vi "Alarms.vi"(0 "Alarm 1":T4, 1 "Alarm 2":T4, 2 "Alarm 3":T4, 3 "Alarm 4":T4, 4 "HW CTRL Data":T2, 5 "Variables State":T3, 7 "error in (no error)":errorcluster) -> (24 "Alarms triggered?":T1, 27 "error out":errorcluster)   [LabVIEW 2014, in "SeqLoop.lvlib"]
doc: "Detecta el estado de las alarmas utilizando el Vi de \"RPNLogicSolverError\"."
uses:
  SeqLoop.lvlib
  TypeDefs/LogicParsedExpression.ctl
  TypeDefs/Variables State.ctl
  TypeDefs/HW CTRL Data.ctl
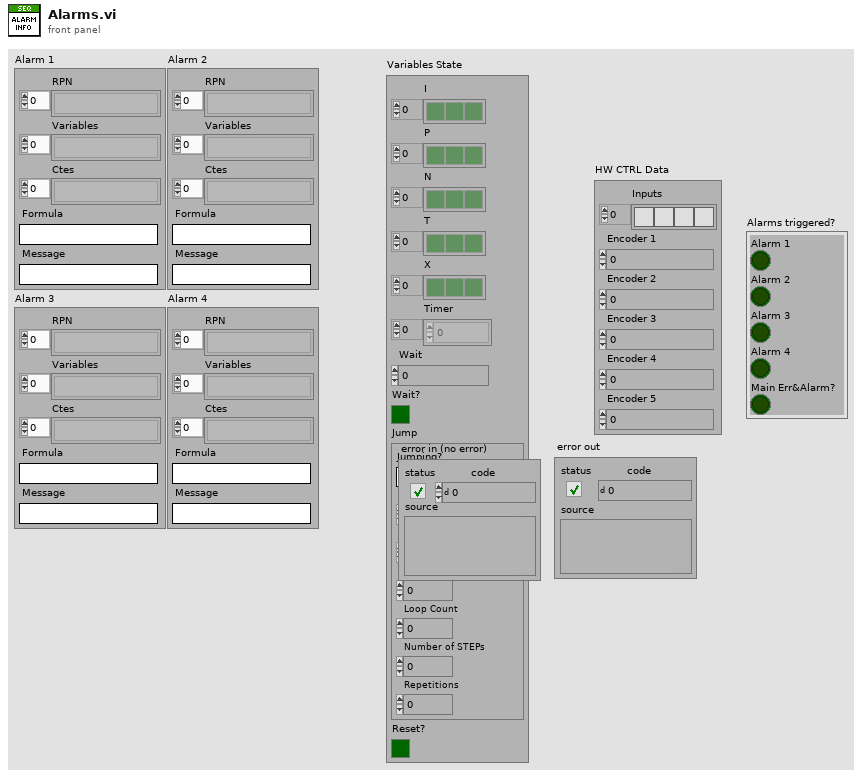
[diagram p1: front panel]
types:
  T1 = cluster{"Alarm 1":bool, "Alarm 2":bool, "Alarm 3":bool, "Alarm 4":bool, "Main Err&Alarm?":bool}
  T2 = typedef "SeqLoop.lvlib/HW CTRL Data.ctl" = cluster{"Inputs":bool[], "Encoder 1":sgl, "Encoder 2":sgl, "Encoder 3":sgl, "Encoder 4":sgl, "Encoder 5":sgl}
  T3 = typedef "SeqLoop.lvlib/Variables State.ctl" = cluster{"I":bool[], "P":bool[], "N":bool[], "T":bool[], "X":bool[], "Timer":u32[], "Wait":u32, "Wait?":bool, "Jump":cluster{"Jumping?":bool, "Previous STEP to Jump":u32, "Initial Jump STEP":u32, "STEP Count":u32, "Loop Count":u32, "Number of STEPs":u32, "Repetitions":u32}, "Reset?":bool}
  T4 = typedef "SeqLoop.lvlib/LogicParsedExpression.ctl" = cluster{"RPN ":string[], "Variables":string[], "Ctes":string[], "Formula":string, "Message":string}
  T5 = cluster{"Logic Result":bool, "Logic Result":bool, "Logic Result":bool, "Logic Result":bool, bool}
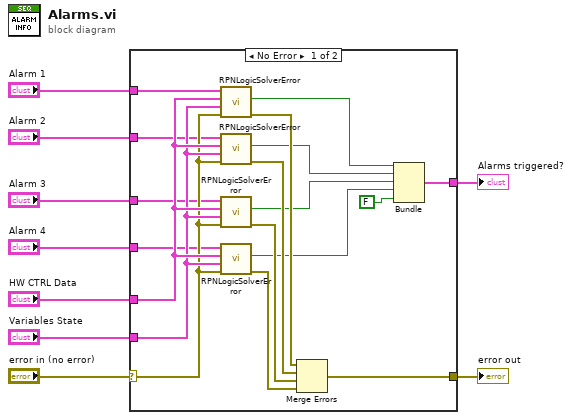
[diagram p0: block diagram]
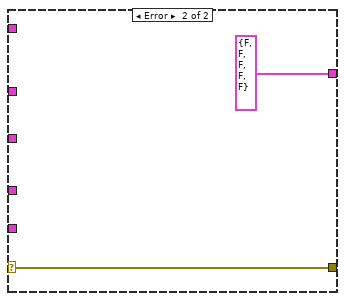
[diagram p2: hidden frame]
diagram:
  n1 = case shown="No Error" "error in (no error)" {
    selector: "error in (no error)" -> [w20 w29]
    tunnel: "Alarm 1" -> [w19 _]
    tunnel: "Alarm 2" -> [w18 _]
    tunnel: "Alarm 3" -> [w17 _]
    tunnel: "Alarm 4" -> [w16 _]
    tunnel: "HW CTRL Data" -> [w27 _]
    tunnel: "Variables State" -> [w26 _]
    tunnel: [w25 w29] -> w2
    tunnel: [w11 T5 {"Logic Result"=FALSE, "Logic Result"=FALSE, "Logic Result"=FALSE, "Logic Result"=FALSE, FALSE}] -> w1
    frame No Error {
      n2 = call "RPNLogicSolverError.vi"("error in"=w20, "Variables State in"=w26, "HW CTRL Data"=w27, "Logic Parsed Expression"=w19) -> ("error out"=w24:errorcluster, "Logic Result"=w15:bool)  [unwired: 5 in, 1 out]
      n3 = call "RPNLogicSolverError.vi"("error in"=w20, "Variables State in"=w26, "HW CTRL Data"=w27, "Logic Parsed Expression"=w18) -> ("error out"=w23:errorcluster, "Logic Result"=w14:bool)  [unwired: 5 in, 1 out]
      n4 = call "RPNLogicSolverError.vi"("error in"=w20, "Variables State in"=w26, "HW CTRL Data"=w27, "Logic Parsed Expression"=w17) -> ("error out"=w22:errorcluster, "Logic Result"=w13:bool)  [unwired: 5 in, 1 out]
      n5 = call "RPNLogicSolverError.vi"("error in"=w20, "Variables State in"=w26, "HW CTRL Data"=w27, "Logic Parsed Expression"=w16) -> ("error out"=w21:errorcluster, "Logic Result"=w12:bool)  [unwired: 5 in, 1 out]
      n6 = Merge Errors(w24, w23, w22, w21) -> (w25:errorcluster)
      n7 = Bundle("Logic Result"=w15, "Logic Result"=w14, "Logic Result"=w13, "Logic Result"=w12, FALSE) -> (w11:T5)  [unwired: 1 in]
    }
    frame Error {
    }
  }
  "error out" <- w2
  "Alarms triggered?" <- w1
